vi "Configure Handler IO Control.vi"(4 "Output 1/ Output 2 Settings (0: High)":u16(ring) items=["High", "Low"], 5 "Port D Direction (0: Input)":u16(ring) items=["Input", "Output"], 6 "Output (1)":i32=1, 7 "Port C Direction (0: Input)":u16(ring) items=["Input", "Output"], 8 "error in (no error)":errorcluster, 9 "Ready For Trigger Signal Output (F: Disable)":bool, 10 "INDEX Signal Output (F: Disable)":bool, 11 "VISA resource name":refnum<visa-resource-name>) -> (0 "error out":errorcluster, 3 "VISA resource name out":refnum<visa-resource-name>)   [LabVIEW 2018, in "Agilent ENA Series.lvlib"]
doc: "Configures the handler IO control settings."
uses:
  Agilent ENA Series.lvlib
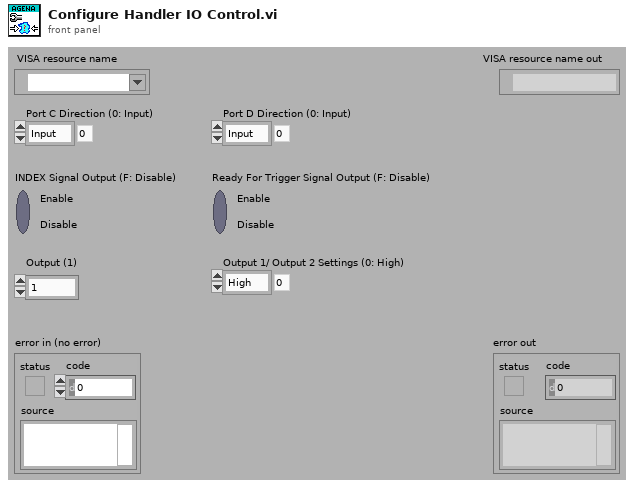
[diagram p1: front panel]
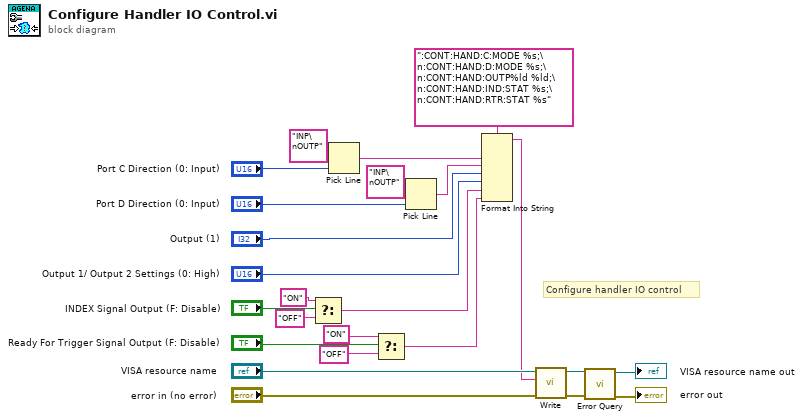
[diagram p0: block diagram]
diagram:
  # "Configure handler IO control"
  n1 = Select(t="ON", s="INDEX Signal Output (F: Disable)", f="OFF") -> (s? t:f=w10:string)
  n2 = Pick Line(multi-line string="INP\nOUTP", line index="Port C Direction (0: Input)") -> (output string=w19:string)  [unwired: 1 in]
  n3 = Select(t="ON", s="Ready For Trigger Signal Output (F: Disable)", f="OFF") -> (s? t:f=w6:string)
  n4 = Pick Line(multi-line string="INP\nOUTP", line index="Port D Direction (0: Input)") -> (output string=w16:string)  [unwired: 1 in]
  n5 = Format Into String(format string=":CONT:HAND:C:MODE %s;\n:CONT:HAND:D:MODE %s;\n:CONT:HAND:OUTP%ld %ld;\n:CONT:HAND:IND:STAT %s;\n:CONT:HAND:RTR:STAT %s", w19, w16, "Output (1)", "Output 1/ Output 2 Settings (0: High)", w10, w6) -> (resulting string=w5:string)  [unwired: 2 in, 1 out]
  n6 = call "Write.vi"("error in (no error)"="error in (no error)", "String ()"=w5, "VISA resource name"="VISA resource name") -> ("error out"=w3:errorcluster, "VISA resource name out"=w4:refnum<visa-resource-name>)  [unwired: 6 in, 1 out]
  n7 = call "Error Query.vi"("error in (no error)"=w3, "VISA resource name"=w4) -> ("error out"=→"error out":errorcluster, "VISA resource name out"=→"VISA resource name out":refnum<visa-resource-name>)  [unwired: 6 in, 2 out]
